vi "Initialize Attributes.vi"(8 "error in (no error)":errorcluster, 10 "Attribute Data":variant, 11 "CS++StartActor in":refnum<class "CS++StartActor.lvclass">) -> (0 "error out":errorcluster, 2 "Found?":bool, 3 "CS++StartActor out":refnum<class "CS++StartActor.lvclass">)   [LabVIEW 2015, in "CS++StartActor.lvlib" / "CS++StartActor.lvclass"]
doc: "Initialize object attribute.\n\nUnique resources should be allocated elsewhere!"
uses:
  CS++StartActor.lvclass
  CS++BaseActor/CS++BaseActor.lvclass/CS++BaseActor.ctl
  CS++StartActor.lvclass/CS++StartActor.ctl
  CS++BaseActor/CS++BaseActor.lvclass
  Classes/CS++BaseClasses/Factory/CS++Factory.lvclass
  Libraries/Utilities/CS++Utilities.lvlib
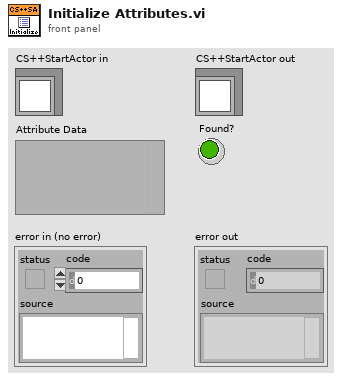
[diagram p1: front panel]
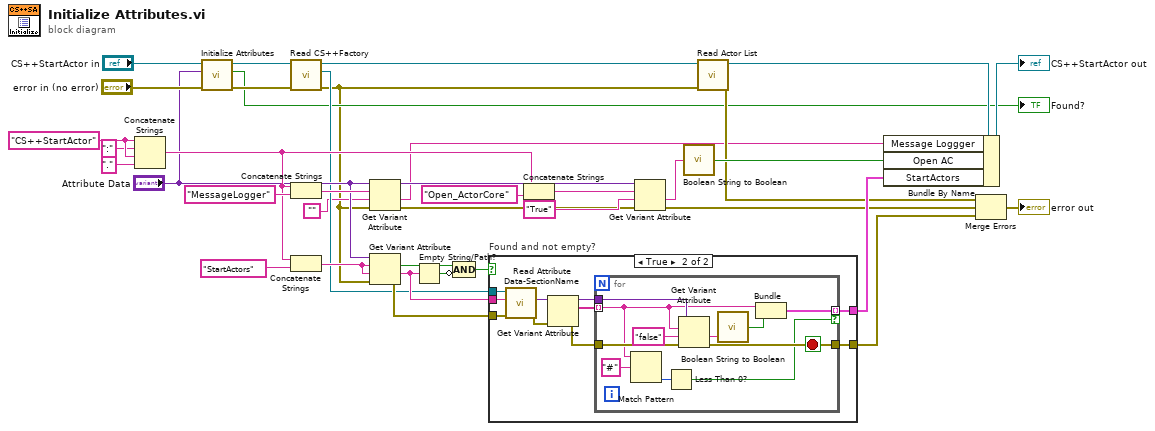
[diagram p0: block diagram]
diagram:
  w37 = "CS++StartActor"
  n1 = Concatenate Strings(w37, ":" ("string"), w37, "." ("string")) -> (w8:string)
  n2 = call-parent "Initialize Attributes.vi"("error in (no error)"="error in (no error)", "Attribute Data"="Attribute Data", "CS++BaseActor in"="CS++StartActor in") -> ("error out"=w24:errorcluster, "Found?"=→"Found?":bool, "CS++BaseActor out"=w25:refnum<class "CS++StartActor.lvclass">)  [unwired: 6 in]
  n3 = call "Read CS++Factory.vi"("error in (no error)"=w24, "CS++BaseActor in"=w25) -> ("error out"=w3:errorcluster, "CS++Factory"=w6:refnum<class "CS++Factory.lvclass">, "CS++BaseActor out"=w13:refnum<class "CS++StartActor.lvclass">)  [unwired: 7 in]
  n4 = Concatenate Strings(w8, "MessageLogger" ("string")) -> (w28:string)
  n5 = Concatenate Strings(w8, "StartActors" ("string")) -> (w19:string)
  n6 = Get Variant Attribute(Variant="Attribute Data", name=w28, default value (empty Variant)="", error in=w3) -> (duplicate Variant=w27:variant, value=w1:string, error out=w2:errorcluster)  [unwired: 1 out]
  n7 = Get Variant Attribute(Variant="Attribute Data", name=w19, default value (empty Variant)=w19, error in=w3) -> (found=w16:bool, value=w17:string, error out=w14:errorcluster)  [unwired: 1 out]
  n8 = Empty String/Path?(string/path=w17) -> (empty?=w18:bool)
  n9 = Compound Arithmetic op=AND(w16, invert w18) -> (w15:bool)
  n10 = case "Found and not empty?" shown="True" w15 {
    tunnel: [w39 w46] -> w10
    tunnel: [_ w45] -> w21
    tunnel: w6 -> [_ w44]
    tunnel: w14 -> [w39 w41]
    tunnel: w17 -> [_ w43]
    frame False {
    }
    frame True {
      n11 = call-dynamic "Read Attribute Data-SectionName.vi"("error in (no error)"=w41, "Object Name"=w43, "CS++Factory in"=w44) -> ("error out"=w40:errorcluster, "Attribute Data"=w42:variant)  [unwired: 6 in, 1 out]
      n12 = Get Variant Attribute(Variant=w42, error in=w40) -> (duplicate Variant=w48:variant, names=w49:string[], error out=w47:errorcluster)  [unwired: 2 in, 1 out]
      n13 = for {
        tunnel: w49 -> [w55] mode=indexing
        tunnel: [w57] -> w45 mode=indexing if=w56
        tunnel: w48 -> [w60]
        tunnel: w47 -> [w59]
        tunnel: [w58] -> w46
        stop <- w58 stop-if-true
        n14 = Match Pattern(string=w55, regular expression="#") -> (offset past match=w50:i32)  [unwired: 1 in, 3 out]
        n15 = Less Than 0?(x=w50) -> (x < 0?=w56:bool)
        n16 = Get Variant Attribute(Variant=w60, name=w55, default value (empty Variant)="false" ("string"), error in=w59) -> (value=w53:string, error out=w58:errorcluster)  [unwired: 2 out]
        n17 = call "Boolean String to Boolean.vi"("T/F String"=w53) -> ("Value"=w52:bool)
        n18 = Bundle(w55, "Value"=w52) -> (w57:cluster{string, "Value":bool})  [unwired: 1 in]
      }
    }
  }
  n19 = Concatenate Strings(w8, "Open_ActorCore" ("string")) -> (w34:string)
  n20 = Get Variant Attribute(Variant=w27, name=w34, default value (empty Variant)="True" ("string"), error in=w2) -> (value=w23:string, error out=w9:errorcluster)  [unwired: 2 out]
  n21 = call "Boolean String to Boolean.vi"("T/F String"=w23) -> ("Value"=w22:bool)
  n22 = call "Read Actor List.vi"("error in (no error)"=w3, "CS++StartActor in"=w13) -> ("error out"=w11:errorcluster, "CS++StartActor out"=w12:refnum<class "CS++StartActor.lvclass">)  [unwired: 8 in]
  n23 = Bundle By Name(cluster=w12, "Message Loggger"=w1, "Open AC"=w22, "StartActors"=w21) -> (→"CS++StartActor out":refnum<class "CS++StartActor.lvclass">)
  n24 = Merge Errors(w11, w9, w10) -> (→"error out":errorcluster)
